vi "Get ControlsTypes.vi"(11 "Ctrls[]":refnum<vi>[](array[refnum])) -> (3 "Controls Refs and Types":T1)   [LabVIEW 2020, in "DQMH_API.lvlib"]
uses:
  DQMH_API.lvlib
  Controls Refs and Type--cluster.ctl
  <vilib>/Utility/Data Type/Type Definitions/Data Type.ctl
  <vilib>/Utility/Data Type/NI_Data Type.lvlib
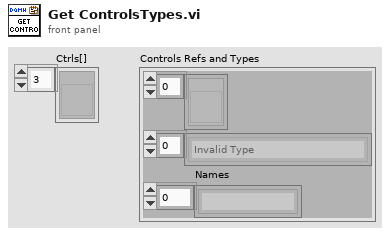
[diagram p1: front panel]
types:
  T1 = typedef "DQMH_API.lvlib/Controls Refs and Type--cluster.ctl" = cluster{"Ctrls Refs ":refnum<vi>[], "Ctrls Types":T2[], "Names":string[]}
  T2 = typedef "NI_Data Type.lvlib/Data Type.ctl" = enum8{"Invalid Type", "Void", "I8", "I16", "I32", "I64", "U8", "U16", "U32", "U64", "Single Float", "Double Float", "Extended Float", "Single Complex", "Double Complex", "Extended Complex", "Enum U8", "Enum U16", "Enum U32", "Enum U64", "Single Float With Unit", "Double Float With Unit", "Extended Float With Unit", "Single Complex with Unit", "Double Complex with Unit", "Extended Complex with Unit", "Boolean", "String", "Path", "Picture", "Tag", "Array", "Cluster", "Variant", "LV Variant", "Waveform", "Timestamp", "Digital Waveform", "Digital Data", "ExpressData", "Refnum", "External Data", "VI", "Poly VI", "LabVIEW Class Instance", "Fixed Point", "Set Collection", "Map Collection"}
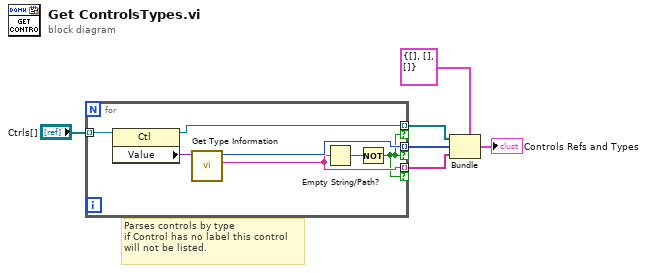
[diagram p0: block diagram]
diagram:
  # "Parses controls by type\nif Control has no label this control\nwill not be listed."
  n1 = for {
    tunnel: "Ctrls[]" -> [w9] mode=indexing
    tunnel: [w10] -> w5 mode=indexing if=w7
    tunnel: [w11] -> w4 mode=indexing if=w7
    tunnel: [w8] -> w1 mode=indexing if=w7
    n2 = property class="Ctl"(reference=w9) -> (reference out=w10:refnum<vi>, "Value"=w12:variant)  [unwired: 1 in, 1 out]
    n3 = call <vilib>:"Get Type Information.vi"("variant"=w12) -> ("name"=w8:string, "type"=w11:T2)  [unwired: 6 in, 3 out]
    n4 = Empty String/Path?(string/path=w8) -> (empty?=w13:bool)
    n5 = Not(x=w13) -> (.not. x?=w7:bool)
  }
  n6 = Bundle(cluster=T1 {"Ctrls Refs "=[], "Ctrls Types"=[], "Names"=[]} ("Indicators"), "Ctrls Refs"=w5, "Ctrls Types"=w4, "Names"=w1) -> (→"Controls Refs and Types":T1)
